vi "PH_Watchdog.set GUI Elements.vi"(0 "VI in":refnum<vi>, 5 "error in":errorcluster) -> (14 "VI out":refnum<vi>, 19 "error out":errorcluster)   [LabVIEW 2014, in "PH_Watchdog.lvlib"]
uses:
  PH_Watchdog.lvlib
  PH_Basics/PH_StatusHandler/PH_StatusHandler.Status.ctl
  PH_Basics/PH_StatusHandler/PH_StatusHandler.lvlib
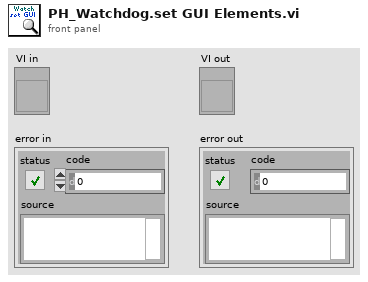
[diagram p1: front panel]
types:
  T1 = typedef "PH_Watchdog.lvlib/PH_Watchdog.i attribute.ctl" = cluster{"GUI Refs":cluster{"All":refnum<vi>, "Failures":refnum<vi>, "Alarms":refnum<vi>, "no info, but linked":refnum<vi>}, "All":T2[]}
  T2 = typedef "PH_Watchdog.lvlib/PH_Watchdog.Dataset.ctl" = cluster{"Instance":string, "Class":string, "Status":T3, "no Link":bool}
  T3 = typedef "PH_StatusHandler.lvlib/PH_StatusHandler.Status.ctl" = i16
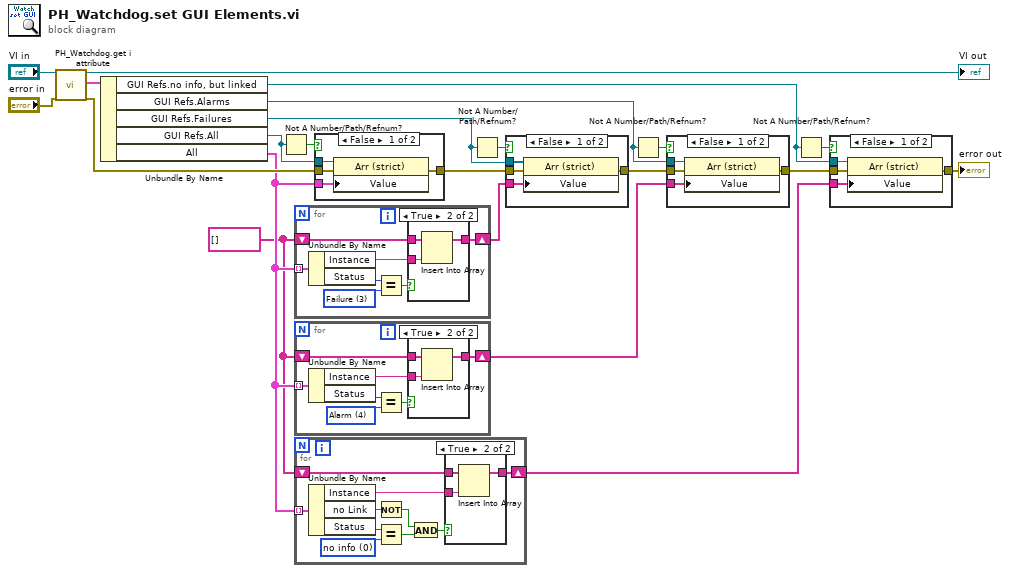
[diagram p0: block diagram]
diagram:
  w6 = string[] []
  n1 = call "PH_Watchdog.get i attribute.vi"("i ref in"="VI in", "error in (no error)"="error in") -> ("i ref out"=→"VI out":refnum<vi>, "i attribute"=w18:T1, "error out"=w20:errorcluster)  [unwired: 15 in]
  n2 = Unbundle By Name(w18) -> ("GUI Refs.no info, but linked"=w1:refnum<vi>, "GUI Refs.Alarms"=w10:refnum<vi>, "GUI Refs.Failures"=w11:refnum<vi>, "GUI Refs.All"=w16:refnum<vi>, "All"=w7:T2[])
  n3 = Not A Number/Path/Refnum?(number/path/refnum=w16) -> (NaN/Path/Refnum?=w17:bool)
  n4 = for {
    tunnel: w7 -> [w26] mode=indexing
    shift-right: [w25] -> w9
    shift-left: w6 -> [w24]
    w28 = T3 3 items=["no info", "off/false/out", "on/true/in", "Failure", "Alarm", "Status 1", "Status 2", "Status 3"] ("y")
    n5 = Unbundle By Name(w26) -> ("Instance"=w23:string, "Status"=w29:T3)
    n6 = Equal?(x=w29, y=w28) -> (x = y?=w27:bool)
    n7 = case shown="True" w27 {
      tunnel: w23 -> [_ w33]
      tunnel: [w30 w32] -> w25
      tunnel: w24 -> [w30 w31]
      frame False {
      }
      frame True {
        n8 = Insert Into Array(array=w31, new element=w33) -> (w32:string[])  [unwired: 1 in]
      }
    }
  }
  n9 = for {
    tunnel: w7 -> [w37] mode=indexing
    shift-right: [w36] -> w8
    shift-left: w6 -> [w35]
    w39 = T3 4 items=["no info", "off/false/out", "on/true/in", "Failure", "Alarm", "Status 1", "Status 2", "Status 3"] ("y")
    n10 = Unbundle By Name(w37) -> ("Instance"=w34:string, "Status"=w40:T3)
    n11 = Equal?(x=w40, y=w39) -> (x = y?=w38:bool)
    n12 = case shown="True" w38 {
      tunnel: w34 -> [_ w44]
      tunnel: [w41 w43] -> w36
      tunnel: w35 -> [w41 w42]
      frame False {
      }
      frame True {
        n13 = Insert Into Array(array=w42, new element=w44) -> (w43:string[])  [unwired: 1 in]
      }
    }
  }
  n14 = for {
    tunnel: w7 -> [w52] mode=indexing
    shift-right: [w51] -> w4
    shift-left: w6 -> [w50]
    w53 = T3 0 items=["no info", "off/false/out", "on/true/in", "Failure", "Alarm", "Status 1", "Status 2", "Status 3"] ("y")
    n15 = Unbundle By Name(w52) -> ("Instance"=w49:string, "no Link"=w48:bool, "Status"=w54:T3)
    n16 = Not(x=w48) -> (.not. x?=w46:bool)
    n17 = Equal?(x=w54, y=w53) -> (x = y?=w45:bool)
    n18 = And(x=w46, y=w45) -> (x .and. y?=w47:bool)
    n19 = case shown="True" w47 {
      tunnel: w49 -> [_ w58]
      tunnel: [w55 w57] -> w51
      tunnel: w50 -> [w55 w56]
      frame False {
      }
      frame True {
        n20 = Insert Into Array(array=w56, new element=w58) -> (w57:string[])  [unwired: 1 in]
      }
    }
  }
  n21 = case shown="False" w17 {
    tunnel: w20 -> [w62 w63]
    tunnel: w7 -> [w61 _]
    tunnel: [w59 w63] -> w13
    tunnel: w16 -> [w60 _]
    frame False {
      n22 = property class="Arr (strict)"(reference=w60, error in=w62, "Value"=w61) -> (error out=w59:errorcluster)  [unwired: 1 out]
    }
    frame True {
    }
  }
  n23 = Not A Number/Path/Refnum?(number/path/refnum=w11) -> (NaN/Path/Refnum?=w15:bool)
  n24 = case shown="False" w15 {
    tunnel: w13 -> [w67 w68]
    tunnel: w9 -> [w66 _]
    tunnel: [w65 w68] -> w12
    tunnel: w11 -> [w64 _]
    frame False {
      n25 = property class="Arr (strict)"(reference=w64, error in=w67, "Value"=w66) -> (error out=w65:errorcluster)  [unwired: 1 out]
    }
    frame True {
    }
  }
  n26 = Not A Number/Path/Refnum?(number/path/refnum=w10) -> (NaN/Path/Refnum?=w14:bool)
  n27 = case shown="False" w14 {
    tunnel: w12 -> [w72 w73]
    tunnel: w8 -> [w71 _]
    tunnel: [w70 w73] -> w3
    tunnel: w10 -> [w69 _]
    frame False {
      n28 = property class="Arr (strict)"(reference=w69, error in=w72, "Value"=w71) -> (error out=w70:errorcluster)  [unwired: 1 out]
    }
    frame True {
    }
  }
  n29 = Not A Number/Path/Refnum?(number/path/refnum=w1) -> (NaN/Path/Refnum?=w5:bool)
  n30 = case shown="False" w5 {
    tunnel: w3 -> [w77 w78]
    tunnel: w4 -> [w76 _]
    tunnel: [w75 w78] -> w2
    tunnel: w1 -> [w74 _]
    frame False {
      n31 = property class="Arr (strict)"(reference=w74, error in=w77, "Value"=w76) -> (error out=w75:errorcluster)  [unwired: 1 out]
    }
    frame True {
    }
  }
  "error out" <- w2
